vi "Get All Pin Names - Cached.vi"(0 "TSM Context in":T1, 1 "Reload Cache?":bool caption="Reload Cache? (F)", 11 "error in":errorcluster) -> (4 "Pin Types":T2[](array[typedef]), 6 "Pin Names":tag[](array[tag]), 15 "error out":errorcluster)   [LabVIEW 2020]
uses:
  TSM Pin Type Identifier.ctl
  <vilib>/NI_TestStand_SemiconductorModule/NI_TestStand_Semiconductor_Module.lvlibp/PinMap/General/SemiconductorModuleContext.ctl
  <vilib>/NI_TestStand_SemiconductorModule/NI_TestStand_Semiconductor_Module.lvlibp
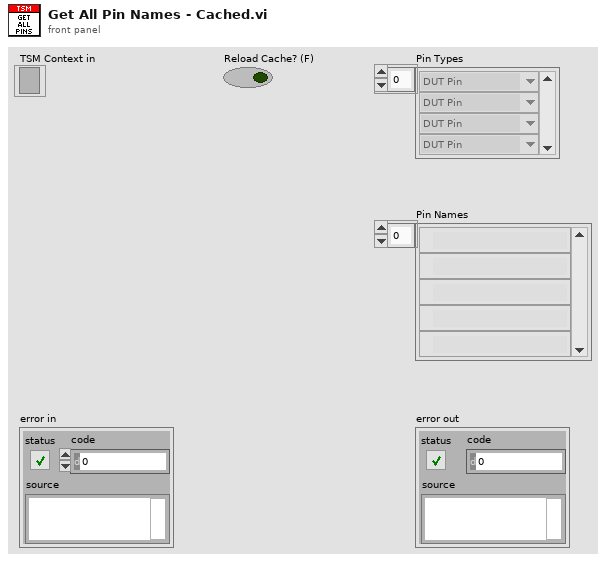
[diagram p1: front panel]
types:
  T1 = typedef "NI_TestStand_Semiconductor_Module.lvlibp/SemiconductorModuleContext.ctl" = refnum<k7>
  T2 = typedef "TSM Pin Type Identifier.ctl" = enum8{"DUT Pin", "System Pin", "Pin Group", "Not Determined"}
  T3 = typedef "NI_TestStand_Semiconductor_Module.lvlibp/TSM_Pin.ctl" = tag
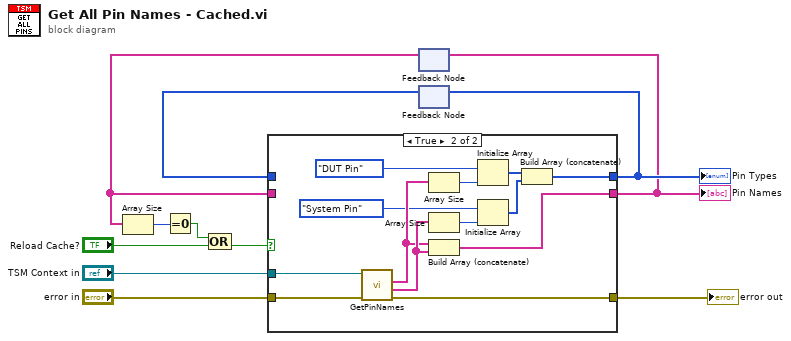
[diagram p0: block diagram]
diagram:
  n1 = feedback #1() -> (w3:T3[])  [unwired: 1 in]
  n2 = Array Size(array=w3) -> (size(s)=w1:i32)
  n3 = Equal To 0?(x=w1) -> (x = 0?=w2:bool)
  n4 = Compound Arithmetic op=OR(w2, "Reload Cache?") -> (w5:bool)
  n5 = feedback #2() -> (w4:T2[])  [unwired: 1 in]
  n6 = case shown="True" w5 {
    tunnel: [w12 w19] -> w6
    tunnel: [w13 w18] -> w7
    tunnel: "TSM Context in" -> [_ w17]
    tunnel: [w14 w16] -> w10
    tunnel: "error in" -> [w14 w15]
    tunnel: w4 -> [w13 _]
    tunnel: w3 -> [w12 _]
    frame False {
    }
    frame True {
      n7 = call <vilib>:"GetPinNames.vi"("error in (no error)"=w15, "Semiconductor Module Context"=w17) -> ("error out"=w16:errorcluster, "System Pins"=w23:T3[], "DUT Pins"=w22:T3[])  [unwired: 6 in, 1 out]
      n8 = Array Size(array=w22) -> (size(s)=w25:i32)
      n9 = Array Size(array=w23) -> (size(s)=w24:i32)
      n10 = Build Array (concatenate)(w22, w23) -> (w19:T3[])
      n11 = Initialize Array(TSM_Pin_Type_Identifier."DUT Pin" ("Enum"), w25) -> (w26:T2[])
      n12 = Initialize Array(TSM_Pin_Type_Identifier."System Pin" ("Enum"), w24) -> (w27:T2[])
      n13 = Build Array (concatenate)(w26, w27) -> (w18:T2[])
    }
  }
  "Pin Names" <- w6
  "Pin Types" <- w7
  "error out" <- w10
  n14 = feedback-in #1(w6) -> ()
  n15 = feedback-in #2(w7) -> ()
